vi "TimerTestsForEXE.vi"(0 "EXE Path":path, 5 "Drona Tests PPL":path, 11 "error in (no error)":errorcluster) -> (15 "error out":errorcluster)   [LabVIEW 2016]
doc: "Run the Drona Tests in EXE"
uses:
  Drona.lvlib
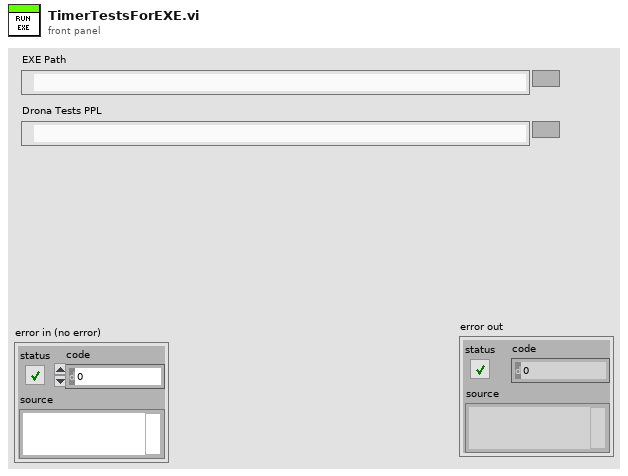
[diagram p1: front panel]
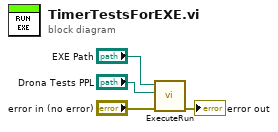
[diagram p0: block diagram]
diagram:
  n1 = call "ExecuteRun.vi"("error in (no error)"="error in (no error)", "Drona Tests PPL"="Drona Tests PPL", "EXE Path"="EXE Path") -> ("error out"=→"error out":errorcluster)  [unwired: 8 in]
